vi "Init Step.vi"(7 "Remove Panel":refnum<user-event>, 8 "error in (no error)":errorcluster, 9 "Update Event":refnum<user-event>, 10 "PanelArray":refnum<class "PanelArray.lvclass">, 11 "Recipe Step in":refnum<class "Recipe Step.lvclass">) -> (0 "error out":errorcluster, 3 "Recipe Step out":refnum<class "Recipe Step.lvclass">)   [LabVIEW 2018, in "Temp Recipe.lvlib" / "Recipe Step.lvclass"]
uses:
  Recipe Step.lvclass
  Libraries/OOPanel/OOPanel/PanelArray/PanelArray.lvclass
  Update Event Data.ctl
  Libraries/OOPanel/OOPanel/Panel/Panel.lvclass
  Recipe Step.lvclass/Recipe Step.ctl
  Temp Recipe.lvlib
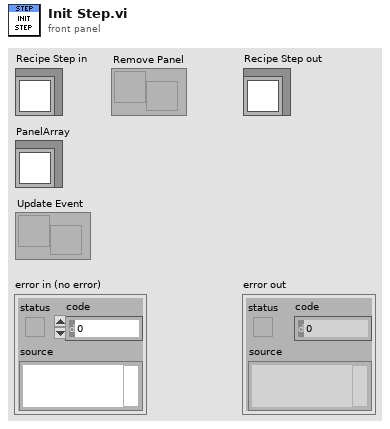
[diagram p1: front panel]
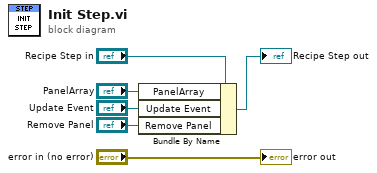
[diagram p0: block diagram]
diagram:
  n1 = Bundle By Name(cluster="Recipe Step in", "PanelArray"="PanelArray", "Update Event"="Update Event", "Remove Panel"="Remove Panel") -> (→"Recipe Step out":refnum<class "Recipe Step.lvclass">)
  "error out" <- "error in (no error)"
